vi "IMAQ subtract background using edges.vi"(8 "error in (no error)":errorcluster, 11 "Image in":T1) -> (1 "Intensity Graph":u16[][](graph), 2 "Line Graph 2":cluster{"x0":sgl, "dx":sgl, "Pixels Line":sgl[]} {"dx" format="%.2f"; "x0" format="%.2f"}, 3 "Refnum out":T1, 4 "Line Graph":cluster{"x0":sgl, "dx":sgl, "Pixels Line":sgl[]} {"dx" format="%.2f"; "x0" format="%.2f"})   [LabVIEW 2020]
uses:
  <vilib>/vision/Image Controls.llb/IMAQ Image.ctl
  <vilib>/Analysis/1siggen.llb/Ramp Pattern by Samples.vi
  <vilib>/vision/NI_Vision_Development_Module.lvlib
  <vilib>/Analysis/NI_AALBase.lvlib
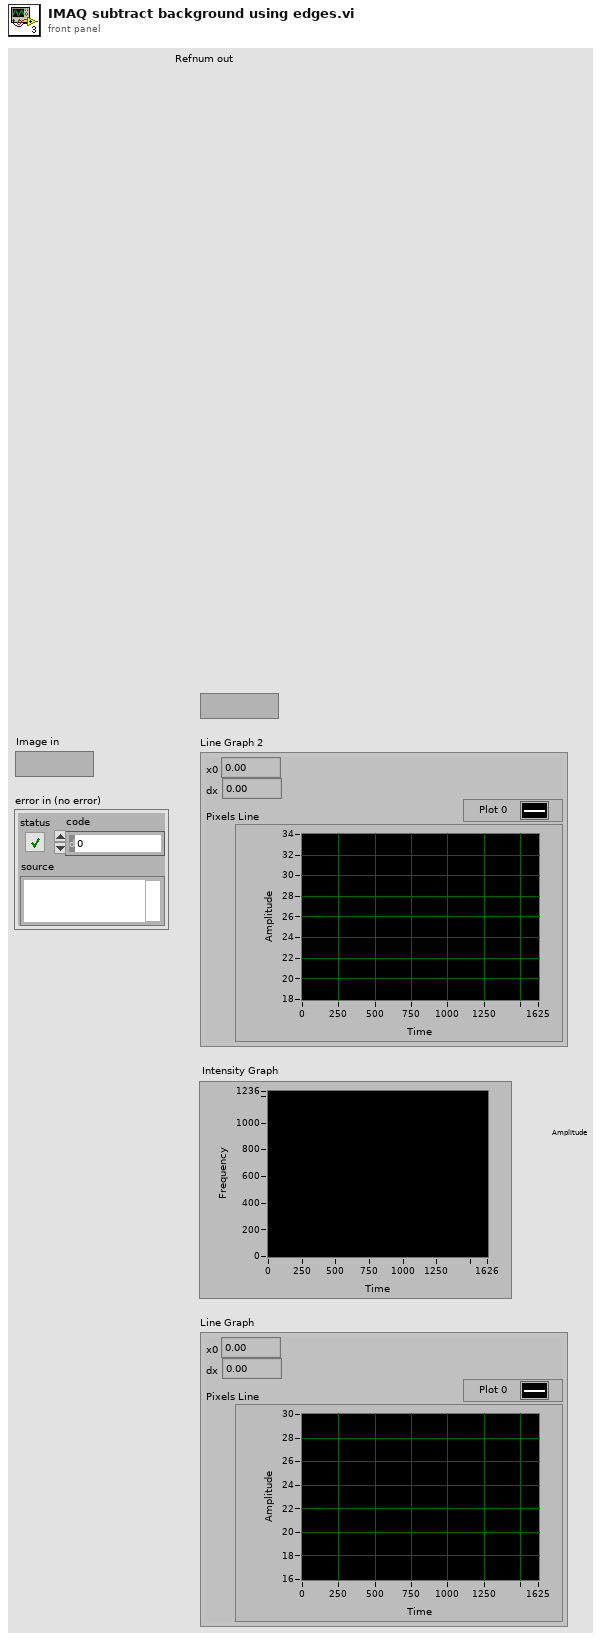
[diagram p1: front panel]
types:
  T1 = typedef "IMAQ Image.ctl" = refnum<image>
  T2 = cluster{"X Size":i32, "Y Size":i32, "% Tolerance":i32}
  T3 = typedef "Image Type" = u32
  T4 = typedef "ROI Descriptor" = cluster{"Global Rectangle":i32[], "Contours":cluster{"ID":enum32{"External", "Internal"}, "Type":u32, "Coordinates":i32[]}[]}
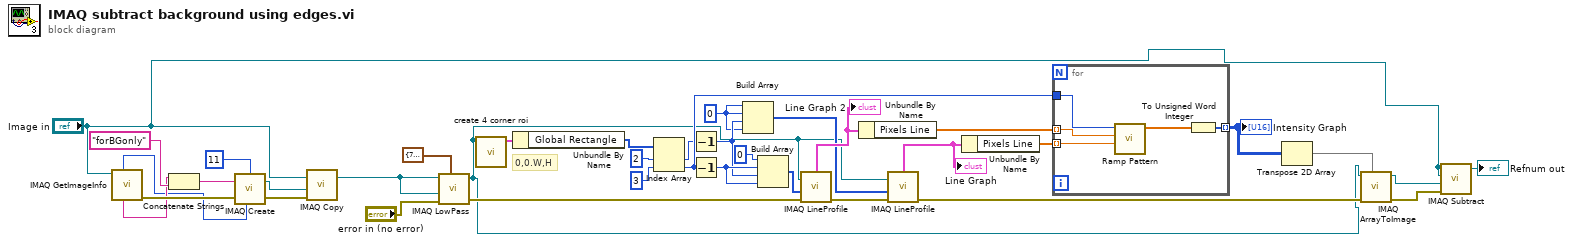
[diagram p0: block diagram]
diagram:
  w12 = 0 ("element")
  # "0,0.W,H"
  n1 = call "IMAQ GetImageInfo"("Image"="Image in") -> ("error out"=w33:errorcluster, "Image Name"=w30:string, "Image Type"=w27:T3)  [unwired: 3 in, 5 out]
  n2 = Concatenate Strings(w30, "forBGonly" ("Image Name")) -> (w28:string)
  n3 = call "IMAQ Create"("Border Size"=11, "Image Name"=w28, "Image Type"=w27, "error in (no error)"=w33) -> ("New Image"=w29:T1, "error out"=w32:errorcluster)  [unwired: 1 in]
  n4 = call "IMAQ Copy"("error in (no error)"=w32, "Image Dst"=w29, "Image Src"="Image in") -> ("Image Dst Out"=w35:T1)  [unwired: 3 in, 1 out]
  n5 = call "IMAQ LowPass"("Image Src"=w35, "Size & Tolerance"=T2 {"X Size"=7, "Y Size"=7, "% Tolerance"=10}, "Image Dst"=w35, "error in (no error)"="error in (no error)") -> ("Image Dst Out"=w1:T1, "error out"=w22:errorcluster)  [unwired: 3 in]
  n6 = call "create 4 corner roi.vi"("Refnum in"=w1) -> ("ROI Descriptor"=w37:T4)  [unwired: 9 in, 1 out]
  n7 = Unbundle By Name(w37) -> ("Global Rectangle"=w3:i32[])
  n8 = Index Array(array=w3, index #1=2 ("index"), index #2=3 ("index")) -> (element #1=w15:i32, element #2=w17:i32)
  n9 = Decrement(x=w15) -> (x-1=w14:i32)
  n10 = Decrement(x=w17) -> (x-1=w16:i32)
  n11 = Build Array(w12, w12, w14, w12) -> (w6:i32[])
  n12 = Build Array(0 ("element"), w16, w14, w16) -> (w7:i32[])
  n13 = call "IMAQ LineProfile"("error in (no error)"=w22, "Line Coordinates"=w7, "Image"=w1) -> ("error out"=w23:errorcluster, "Line Graph"=w9:cluster{"x0":sgl, "dx":sgl, "Pixels Line":sgl[]})  [unwired: 2 in, 2 out]
  "Line Graph 2" <- w9
  n14 = Unbundle By Name(w9) -> ("Pixels Line"=w11:sgl[])
  n15 = call "IMAQ LineProfile"("error in (no error)"=w23, "Line Coordinates"=w6, "Image"=w1) -> ("error out"=w24:errorcluster, "Line Graph"=w8:cluster{"x0":sgl, "dx":sgl, "Pixels Line":sgl[]})  [unwired: 2 in, 2 out]
  "Line Graph" <- w8
  n16 = Unbundle By Name(w8) -> ("Pixels Line"=w10:sgl[])
  n17 = for {
    tunnel: w10 -> [w40] mode=indexing
    tunnel: w11 -> [w41] mode=indexing
    tunnel: w17 -> [w42]
    tunnel: [w38] -> w18 mode=indexing
    n18 = call-poly <vilib>:"Ramp Pattern.vi"("start"=w40, "end"=w41, "samples"=w42) -> ("Ramp Pattern"=w39:dbl[])  [unwired: 7 in, 1 out]
    n19 = To Unsigned Word Integer(number=w39) -> (unsigned 16bit integer=w38:u16[])
  }
  "Intensity Graph" <- w18
  n20 = Transpose 2D Array(2D array=w18) -> (transposed array=w19:u16[][])
  n21 = call "IMAQ ArrayToImage"("Image Pixels (U16)"=w19, "error in (no error)"=w24, "Image"=w1) -> ("error out"=w25:errorcluster, "Image Out"=w21:T1)  [unwired: 7 in]
  n22 = call "IMAQ Subtract"("Image Src A"="Image in", "Image Dst"="Image in", "Image Src B"=w21, "error in (no error)"=w25) -> ("Image Dst Out"=→"Refnum out":T1)  [unwired: 3 in, 1 out]
